vi "main(Test DQMH modules).vi"() -> ()   [LabVIEW 2018, in "Application.lvlib"] (continued)
        n3446 = Not(x=w8018) -> (.not. x?=w8015:bool)
        n3447 = Or(x=w8017, y=w8015) -> (x .or. y?=w8016:bool)
        n3448 = case shown="False" w8016 {
          tunnel: [w8045 _] -> w8027
          tunnel: w8024 -> [w8044 _]
          frame False {
            w8033 = T9 {"command"="", "data"=variant} ("element")
            w8032 = "MEAS.mux6_1"
            n3449 = To Variant(anything=T2."mux6_1_channel3_3" ("mux6_1(3wires)_encode")) -> (Variant=w8042:variant)
            n3450 = To Variant(anything=T2."mux6_1_channel3_2" ("mux6_1(3wires)_encode")) -> (Variant=w8040:variant)
            n3451 = Bundle By Name(cluster=w8033, "command"=w8032, "data"=w8040) -> (w8039:T9)
            n3452 = Bundle By Name(cluster=w8033, "command"=w8032, "data"=w8042) -> (w8038:T9)
            n3453 = Bundle By Name(cluster=w8033, "command"="MEAS.DMM dual read") -> (w8036:T9)
            n3454 = Build Array(w8039, w8038, w8036) -> (w8034:T9[])
            n3455 = Reverse 1D Array(array=w8034) -> (reversed array=w8035:T9[])
            n3456 = for {
              tunnel: [w8051] -> w8045 mode=indexing
              tunnel: w8044 -> [w8050]
              tunnel: w8035 -> [w8049] mode=indexing
              n3457 = Unbundle By Name(w8049) -> ("command"=w8048:string, "data"=w8047:variant)
              n3458 = call "App enquece.vi"("Priority Enquece"=TRUE, "command data"=w8047, "command"=w8048, "queue in"=w8050) -> ("error out"=w8051:errorcluster)  [unwired: 6 in, 1 out]
            }
          }
          frame True {
          }
        }
        n3459 = Merge Errors(w8025, w8027) -> (w8026:errorcluster)
      }
      frame "Test DRV 16" {
        w8061 = 16  # DUT index(1-60)
        n3460 = disable-structure shown="LOGGING==TRUE" {
          disable-tunnel: w8062 -> [w8094 _]
          frame condition #0 (active) {
            n3461 = Empty String/Path?(string/path=w8094) -> (empty?=w8096:bool)
            n3462 = Select(t="Quece timeout", s=w8096, f=w8094) -> (s? t:f=w8093:string)
            n3463 = call "string log (SubVI).vi"("state Name"=w8093) -> ()  [unwired: 9 in, 2 out]
          }
          frame condition #1 {
          }
        }
        n3464 = call "progress string(SubVI).vi"("String 3"=w8062, "String in"=w8063) -> ("String out"=w8064:string)  [unwired: 9 in]
        n3465 = call "FGV DRV stand.vi"() -> ("Sub-Test.DCV"=w8060:bool)  [unwired: 10 in, 1 out]
        n3466 = call "FGV Driver Data.vi"("DUT index(1-60)"=w8061) -> ("DUT SC"=w8059:bool)  [unwired: 7 in, 3 out]
        n3467 = Not(x=w8060) -> (.not. x?=w8056:bool)
        n3468 = Or(x=w8059, y=w8056) -> (x .or. y?=w8058:bool)
        n3469 = case shown="False" w8058 {
          tunnel: [w8086 _] -> w8068
          tunnel: w8066 -> [w8085 _]
          frame False {
            w8074 = T9 {"command"="", "data"=variant} ("element")
            w8073 = "MEAS.mux6_1"
            n3470 = To Variant(anything=T2."mux6_1_channel4_3" ("mux6_1(3wires)_encode")) -> (Variant=w8083:variant)
            n3471 = To Variant(anything=T2."mux6_1_channel4_2" ("mux6_1(3wires)_encode")) -> (Variant=w8081:variant)
            n3472 = Bundle By Name(cluster=w8074, "command"=w8073, "data"=w8081) -> (w8080:T9)
            n3473 = Bundle By Name(cluster=w8074, "command"=w8073, "data"=w8083) -> (w8079:T9)
            n3474 = Bundle By Name(cluster=w8074, "command"="MEAS.DMM dual read") -> (w8077:T9)
            n3475 = Build Array(w8080, w8079, w8077) -> (w8075:T9[])
            n3476 = Reverse 1D Array(array=w8075) -> (reversed array=w8076:T9[])
            n3477 = for {
              tunnel: [w8092] -> w8086 mode=indexing
              tunnel: w8085 -> [w8091]
              tunnel: w8076 -> [w8090] mode=indexing
              n3478 = Unbundle By Name(w8090) -> ("command"=w8089:string, "data"=w8088:variant)
              n3479 = call "App enquece.vi"("Priority Enquece"=TRUE, "command data"=w8088, "command"=w8089, "queue in"=w8091) -> ("error out"=w8092:errorcluster)  [unwired: 6 in, 1 out]
            }
          }
          frame True {
          }
        }
        n3480 = Merge Errors(w8067, w8068) -> (w8057:errorcluster)
      }
      frame "Test DRV 17" {
        w8101 = 17  # DUT index(1-60)
        n3481 = disable-structure shown="LOGGING==TRUE" {
          disable-tunnel: w8102 -> [w8135 _]
          frame condition #0 (active) {
            n3482 = Empty String/Path?(string/path=w8135) -> (empty?=w8137:bool)
            n3483 = Select(t="Quece timeout", s=w8137, f=w8135) -> (s? t:f=w8134:string)
            n3484 = call "string log (SubVI).vi"("state Name"=w8134) -> ()  [unwired: 9 in, 2 out]
          }
          frame condition #1 {
          }
        }
        n3485 = call "progress string(SubVI).vi"("String 3"=w8102, "String in"=w8103) -> ("String out"=w8104:string)  [unwired: 9 in]
        n3486 = call "FGV DRV stand.vi"() -> ("Sub-Test.DCV"=w8100:bool)  [unwired: 10 in, 1 out]
        n3487 = call "FGV Driver Data.vi"("DUT index(1-60)"=w8101) -> ("DUT SC"=w8099:bool)  [unwired: 7 in, 3 out]
        n3488 = Not(x=w8100) -> (.not. x?=w8097:bool)
        n3489 = Or(x=w8099, y=w8097) -> (x .or. y?=w8098:bool)
        n3490 = case shown="False" w8098 {
          tunnel: [w8127 _] -> w8109
          tunnel: w8106 -> [w8126 _]
          frame False {
            w8115 = T9 {"command"="", "data"=variant} ("element")
            w8114 = "MEAS.mux6_1"
            n3491 = To Variant(anything=T2."mux6_1_channel5_3" ("mux6_1(3wires)_encode")) -> (Variant=w8124:variant)
            n3492 = To Variant(anything=T2."mux6_1_channel5_2" ("mux6_1(3wires)_encode")) -> (Variant=w8122:variant)
            n3493 = Bundle By Name(cluster=w8115, "command"=w8114, "data"=w8122) -> (w8121:T9)
            n3494 = Bundle By Name(cluster=w8115, "command"=w8114, "data"=w8124) -> (w8120:T9)
            n3495 = Bundle By Name(cluster=w8115, "command"="MEAS.DMM dual read") -> (w8118:T9)
            n3496 = Build Array(w8121, w8120, w8118) -> (w8116:T9[])
            n3497 = Reverse 1D Array(array=w8116) -> (reversed array=w8117:T9[])
            n3498 = for {
              tunnel: [w8133] -> w8127 mode=indexing
              tunnel: w8126 -> [w8132]
              tunnel: w8117 -> [w8131] mode=indexing
              n3499 = Unbundle By Name(w8131) -> ("command"=w8130:string, "data"=w8129:variant)
              n3500 = call "App enquece.vi"("Priority Enquece"=TRUE, "command data"=w8129, "command"=w8130, "queue in"=w8132) -> ("error out"=w8133:errorcluster)  [unwired: 6 in, 1 out]
            }
          }
          frame True {
          }
        }
        n3501 = Merge Errors(w8107, w8109) -> (w8108:errorcluster)
      }
      frame "Test DRV 18" {
        w8145 = 18  # DUT index(1-60)
        n3502 = disable-structure shown="LOGGING==TRUE" {
          disable-tunnel: w8142 -> [w8176 _]
          frame condition #0 (active) {
            n3503 = Empty String/Path?(string/path=w8176) -> (empty?=w8178:bool)
            n3504 = Select(t="Quece timeout", s=w8178, f=w8176) -> (s? t:f=w8175:string)
            n3505 = call "string log (SubVI).vi"("state Name"=w8175) -> ()  [unwired: 9 in, 2 out]
          }
          frame condition #1 {
          }
        }
        n3506 = call "progress string(SubVI).vi"("String 3"=w8142, "String in"=w8143) -> ("String out"=w8144:string)  [unwired: 9 in]
        n3507 = call "FGV DRV stand.vi"() -> ("Sub-Test.DCV"=w8139:bool)  [unwired: 10 in, 1 out]
        n3508 = call "FGV Driver Data.vi"("DUT index(1-60)"=w8145) -> ("DUT SC"=w8140:bool)  [unwired: 7 in, 3 out]
        n3509 = Not(x=w8139) -> (.not. x?=w8138:bool)
        n3510 = Or(x=w8140, y=w8138) -> (x .or. y?=w8141:bool)
        n3511 = case shown="False" w8141 {
          tunnel: [w8168 _] -> w8150
          tunnel: w8147 -> [w8167 _]
          frame False {
            w8156 = T9 {"command"="", "data"=variant} ("element")
            w8155 = "MEAS.mux6_1"
            n3512 = To Variant(anything=T2."mux6_1_channel6_3" ("mux6_1(3wires)_encode")) -> (Variant=w8165:variant)
            n3513 = To Variant(anything=T2."mux6_1_channel6_2" ("mux6_1(3wires)_encode")) -> (Variant=w8163:variant)
            n3514 = Bundle By Name(cluster=w8156, "command"=w8155, "data"=w8163) -> (w8162:T9)
            n3515 = Bundle By Name(cluster=w8156, "command"=w8155, "data"=w8165) -> (w8161:T9)
            n3516 = Bundle By Name(cluster=w8156, "command"="MEAS.DMM dual read") -> (w8159:T9)
            n3517 = Build Array(w8162, w8161, w8159) -> (w8157:T9[])
            n3518 = Reverse 1D Array(array=w8157) -> (reversed array=w8158:T9[])
            n3519 = for {
              tunnel: [w8174] -> w8168 mode=indexing
              tunnel: w8167 -> [w8173]
              tunnel: w8158 -> [w8172] mode=indexing
              n3520 = Unbundle By Name(w8172) -> ("command"=w8171:string, "data"=w8170:variant)
              n3521 = call "App enquece.vi"("Priority Enquece"=TRUE, "command data"=w8170, "command"=w8171, "queue in"=w8173) -> ("error out"=w8174:errorcluster)  [unwired: 6 in, 1 out]
            }
          }
          frame True {
          }
        }
        n3522 = Merge Errors(w8148, w8150) -> (w8149:errorcluster)
      }
      frame "Test DRV 19" {
        w8183 = 19  # DUT index(1-60)
        n3523 = disable-structure shown="LOGGING==TRUE" {
          disable-tunnel: w8184 -> [w8217 _]
          frame condition #0 (active) {
            n3524 = Empty String/Path?(string/path=w8217) -> (empty?=w8219:bool)
            n3525 = Select(t="Quece timeout", s=w8219, f=w8217) -> (s? t:f=w8216:string)
            n3526 = call "string log (SubVI).vi"("state Name"=w8216) -> ()  [unwired: 9 in, 2 out]
          }
          frame condition #1 {
          }
        }
        n3527 = call "progress string(SubVI).vi"("String 3"=w8184, "String in"=w8185) -> ("String out"=w8186:string)  [unwired: 9 in]
        n3528 = call "FGV Driver Data.vi"("DUT index(1-60)"=w8183) -> ("DUT SC"=w8181:bool)  [unwired: 7 in, 3 out]
        n3529 = call "FGV DRV stand.vi"() -> ("Sub-Test.DCV"=w8180:bool)  [unwired: 10 in, 1 out]
        n3530 = Not(x=w8180) -> (.not. x?=w8179:bool)
        n3531 = Or(x=w8181, y=w8179) -> (x .or. y?=w8182:bool)
        n3532 = case shown="False" w8182 {
          tunnel: [w8209 _] -> w8191
          tunnel: w8188 -> [w8208 _]
          frame False {
            w8197 = T9 {"command"="", "data"=variant} ("element")
            w8196 = "MEAS.mux6_1"
            n3533 = To Variant(anything=T2."mux6_1_channel1_3" ("mux6_1(3wires)_encode")) -> (Variant=w8206:variant)
            n3534 = To Variant(anything=T2."mux6-1_channel1_2" ("mux6_1(3wires)_encode")) -> (Variant=w8204:variant)
            n3535 = Bundle By Name(cluster=w8197, "command"=w8196, "data"=w8204) -> (w8203:T9)
            n3536 = Bundle By Name(cluster=w8197, "command"=w8196, "data"=w8206) -> (w8202:T9)
            n3537 = Bundle By Name(cluster=w8197, "command"="MEAS.DMM dual read") -> (w8200:T9)
            n3538 = Build Array(w8203, w8202, w8200) -> (w8198:T9[])
            n3539 = Reverse 1D Array(array=w8198) -> (reversed array=w8199:T9[])
            n3540 = for {
              tunnel: [w8215] -> w8209 mode=indexing
              tunnel: w8208 -> [w8214]
              tunnel: w8199 -> [w8213] mode=indexing
              n3541 = Unbundle By Name(w8213) -> ("command"=w8212:string, "data"=w8211:variant)
              n3542 = call "App enquece.vi"("Priority Enquece"=TRUE, "command data"=w8211, "command"=w8212, "queue in"=w8214) -> ("error out"=w8215:errorcluster)  [unwired: 6 in, 1 out]
            }
          }
          frame True {
          }
        }
        n3543 = Merge Errors(w8189, w8191) -> (w8190:errorcluster)
      }
      frame "Test DRV 20" {
        w8224 = 20  # DUT index(1-60)
        n3544 = call "progress string(SubVI).vi"("String 3"=w8225, "String in"=w8226) -> ("String out"=w8227:string)  [unwired: 9 in]
        n3545 = disable-structure shown="LOGGING==TRUE" {
          disable-tunnel: w8225 -> [w8258 _]
          frame condition #0 (active) {
            n3546 = Empty String/Path?(string/path=w8258) -> (empty?=w8260:bool)
            n3547 = Select(t="Quece timeout", s=w8260, f=w8258) -> (s? t:f=w8257:string)
            n3548 = call "string log (SubVI).vi"("state Name"=w8257) -> ()  [unwired: 9 in, 2 out]
          }
          frame condition #1 {
          }
        }
        n3549 = call "FGV DRV stand.vi"() -> ("Sub-Test.DCV"=w8223:bool)  [unwired: 10 in, 1 out]
        n3550 = call "FGV Driver Data.vi"("DUT index(1-60)"=w8224) -> ("DUT SC"=w8222:bool)  [unwired: 7 in, 3 out]
        n3551 = Not(x=w8223) -> (.not. x?=w8220:bool)
        n3552 = Or(x=w8222, y=w8220) -> (x .or. y?=w8221:bool)
        n3553 = case shown="False" w8221 {
          tunnel: [w8250 _] -> w8232
          tunnel: w8229 -> [w8249 _]
          frame False {
            w8238 = T9 {"command"="", "data"=variant} ("element")
            w8237 = "MEAS.mux6_1"
            n3554 = To Variant(anything=T2."mux6_1_channel2_3" ("mux6_1(3wires)_encode")) -> (Variant=w8247:variant)
            n3555 = To Variant(anything=T2."mux6_1_channel2_2" ("mux6_1(3wires)_encode")) -> (Variant=w8245:variant)
            n3556 = Bundle By Name(cluster=w8238, "command"=w8237, "data"=w8245) -> (w8244:T9)
            n3557 = Bundle By Name(cluster=w8238, "command"=w8237, "data"=w8247) -> (w8243:T9)
            n3558 = Bundle By Name(cluster=w8238, "command"="MEAS.DMM dual read") -> (w8241:T9)
            n3559 = Build Array(w8244, w8243, w8241) -> (w8239:T9[])
            n3560 = Reverse 1D Array(array=w8239) -> (reversed array=w8240:T9[])
            n3561 = for {
              tunnel: [w8256] -> w8250 mode=indexing
              tunnel: w8249 -> [w8255]
              tunnel: w8240 -> [w8254] mode=indexing
              n3562 = Unbundle By Name(w8254) -> ("command"=w8253:string, "data"=w8252:variant)
              n3563 = call "App enquece.vi"("Priority Enquece"=TRUE, "command data"=w8252, "command"=w8253, "queue in"=w8255) -> ("error out"=w8256:errorcluster)  [unwired: 6 in, 1 out]
            }
          }
          frame True {
          }
        }
        n3564 = Merge Errors(w8230, w8232) -> (w8231:errorcluster)
      }
      frame "Test DRV 21" {
        w8266 = 21  # DUT index(1-60)
        n3565 = call "progress string(SubVI).vi"("String 3"=w8267, "String in"=w8268) -> ("String out"=w8269:string)  [unwired: 9 in]
        n3566 = disable-structure shown="LOGGING==TRUE" {
          disable-tunnel: w8267 -> [w8299 _]
          frame condition #0 (active) {
            n3567 = Empty String/Path?(string/path=w8299) -> (empty?=w8301:bool)
            n3568 = Select(t="Quece timeout", s=w8301, f=w8299) -> (s? t:f=w8298:string)
            n3569 = call "string log (SubVI).vi"("state Name"=w8298) -> ()  [unwired: 9 in, 2 out]
          }
          frame condition #1 {
          }
        }
        n3570 = call "FGV DRV stand.vi"() -> ("Sub-Test.DCV"=w8264:bool)  [unwired: 10 in, 1 out]
        n3571 = call "FGV Driver Data.vi"("DUT index(1-60)"=w8266) -> ("DUT SC"=w8263:bool)  [unwired: 7 in, 3 out]
        n3572 = Not(x=w8264) -> (.not. x?=w8261:bool)
        n3573 = Or(x=w8263, y=w8261) -> (x .or. y?=w8262:bool)
        n3574 = case shown="False" w8262 {
          tunnel: [w8291 _] -> w8273
          tunnel: w8271 -> [w8290 _]
          frame False {
            w8279 = T9 {"command"="", "data"=variant} ("element")
            w8278 = "MEAS.mux6_1"
            n3575 = To Variant(anything=T2."mux6_1_channel3_2" ("mux6_1(3wires)_encode")) -> (Variant=w8286:variant)
            n3576 = To Variant(anything=T2."mux6_1_channel3_3" ("mux6_1(3wires)_encode")) -> (Variant=w8288:variant)
            n3577 = Bundle By Name(cluster=w8279, "command"=w8278, "data"=w8286) -> (w8285:T9)
            n3578 = Bundle By Name(cluster=w8279, "command"=w8278, "data"=w8288) -> (w8284:T9)
            n3579 = Bundle By Name(cluster=w8279, "command"="MEAS.DMM dual read") -> (w8282:T9)
            n3580 = Build Array(w8285, w8284, w8282) -> (w8280:T9[])
            n3581 = Reverse 1D Array(array=w8280) -> (reversed array=w8281:T9[])
            n3582 = for {
              tunnel: [w8297] -> w8291 mode=indexing
              tunnel: w8290 -> [w8296]
              tunnel: w8281 -> [w8295] mode=indexing
              n3583 = Unbundle By Name(w8295) -> ("command"=w8294:string, "data"=w8293:variant)
              n3584 = call "App enquece.vi"("Priority Enquece"=TRUE, "command data"=w8293, "command"=w8294, "queue in"=w8296) -> ("error out"=w8297:errorcluster)  [unwired: 6 in, 1 out]
            }
          }
          frame True {
          }
        }
        n3585 = Merge Errors(w8272, w8273) -> (w8265:errorcluster)
      }
      frame "Test DRV 22" {
        w8306 = 22  # DUT index(1-60)
        n3586 = disable-structure shown="LOGGING==TRUE" {
          disable-tunnel: w8307 -> [w8340 _]
          frame condition #0 (active) {
            n3587 = Empty String/Path?(string/path=w8340) -> (empty?=w8342:bool)
            n3588 = Select(t="Quece timeout", s=w8342, f=w8340) -> (s? t:f=w8339:string)
            n3589 = call "string log (SubVI).vi"("state Name"=w8339) -> ()  [unwired: 9 in, 2 out]
          }
          frame condition #1 {
          }
        }
        n3590 = call "progress string(SubVI).vi"("String 3"=w8307, "String in"=w8308) -> ("String out"=w8309:string)  [unwired: 9 in]
        n3591 = call "FGV DRV stand.vi"() -> ("Sub-Test.DCV"=w8305:bool)  [unwired: 10 in, 1 out]
        n3592 = call "FGV Driver Data.vi"("DUT index(1-60)"=w8306) -> ("DUT SC"=w8304:bool)  [unwired: 7 in, 3 out]
        n3593 = Not(x=w8305) -> (.not. x?=w8302:bool)
        n3594 = Or(x=w8304, y=w8302) -> (x .or. y?=w8303:bool)
        n3595 = case shown="False" w8303 {
          tunnel: [w8332 _] -> w8314
          tunnel: w8311 -> [w8331 _]
          frame False {
            w8320 = T9 {"command"="", "data"=variant} ("element")
            w8319 = "MEAS.mux6_1"
            n3596 = To Variant(anything=T2."mux6_1_channel4_2" ("mux6_1(3wires)_encode")) -> (Variant=w8327:variant)
            n3597 = To Variant(anything=T2."mux6_1_channel4_3" ("mux6_1(3wires)_encode")) -> (Variant=w8329:variant)
            n3598 = Bundle By Name(cluster=w8320, "command"=w8319, "data"=w8327) -> (w8326:T9)
            n3599 = Bundle By Name(cluster=w8320, "command"=w8319, "data"=w8329) -> (w8325:T9)
            n3600 = Bundle By Name(cluster=w8320, "command"="MEAS.DMM dual read") -> (w8323:T9)
            n3601 = Build Array(w8326, w8325, w8323) -> (w8321:T9[])
            n3602 = Reverse 1D Array(array=w8321) -> (reversed array=w8322:T9[])
            n3603 = for {
              tunnel: [w8338] -> w8332 mode=indexing
              tunnel: w8331 -> [w8337]
              tunnel: w8322 -> [w8336] mode=indexing
              n3604 = Unbundle By Name(w8336) -> ("command"=w8335:string, "data"=w8334:variant)
              n3605 = call "App enquece.vi"("Priority Enquece"=TRUE, "command data"=w8334, "command"=w8335, "queue in"=w8337) -> ("error out"=w8338:errorcluster)  [unwired: 6 in, 1 out]
            }
          }
          frame True {
          }
        }
        n3606 = Merge Errors(w8312, w8314) -> (w8313:errorcluster)
      }
      frame "Test DRV 23" {
        w8348 = 23  # DUT index(1-60)
        n3607 = call "progress string(SubVI).vi"("String 3"=w8349, "String in"=w8350) -> ("String out"=w8351:string)  [unwired: 9 in]
        n3608 = disable-structure shown="LOGGING==TRUE" {
          disable-tunnel: w8349 -> [w8381 _]
          frame condition #0 (active) {
            n3609 = Empty String/Path?(string/path=w8381) -> (empty?=w8383:bool)
            n3610 = Select(t="Quece timeout", s=w8383, f=w8381) -> (s? t:f=w8380:string)
            n3611 = call "string log (SubVI).vi"("state Name"=w8380) -> ()  [unwired: 9 in, 2 out]
          }
          frame condition #1 {
          }
        }
        n3612 = call "FGV DRV stand.vi"() -> ("Sub-Test.DCV"=w8346:bool)  [unwired: 10 in, 1 out]
        n3613 = call "FGV Driver Data.vi"("DUT index(1-60)"=w8348) -> ("DUT SC"=w8345:bool)  [unwired: 7 in, 3 out]
        n3614 = Not(x=w8346) -> (.not. x?=w8343:bool)
        n3615 = Or(x=w8345, y=w8343) -> (x .or. y?=w8344:bool)
        n3616 = case shown="False" w8344 {
          tunnel: [w8373 _] -> w8355
          tunnel: w8353 -> [w8372 _]
          frame False {
            w8361 = T9 {"command"="", "data"=variant} ("element")
            w8360 = "MEAS.mux6_1"
            n3617 = To Variant(anything=T2."mux6_1_channel5_3" ("mux6_1(3wires)_encode")) -> (Variant=w8370:variant)
            n3618 = To Variant(anything=T2."mux6_1_channel5_2" ("mux6_1(3wires)_encode")) -> (Variant=w8368:variant)
            n3619 = Bundle By Name(cluster=w8361, "command"=w8360, "data"=w8368) -> (w8367:T9)
            n3620 = Bundle By Name(cluster=w8361, "command"=w8360, "data"=w8370) -> (w8366:T9)
            n3621 = Bundle By Name(cluster=w8361, "command"="MEAS.DMM dual read") -> (w8364:T9)
            n3622 = Build Array(w8367, w8366, w8364) -> (w8362:T9[])
            n3623 = Reverse 1D Array(array=w8362) -> (reversed array=w8363:T9[])
            n3624 = for {
              tunnel: [w8379] -> w8373 mode=indexing
              tunnel: w8372 -> [w8378]
              tunnel: w8363 -> [w8377] mode=indexing
              n3625 = Unbundle By Name(w8377) -> ("command"=w8376:string, "data"=w8375:variant)
              n3626 = call "App enquece.vi"("Priority Enquece"=TRUE, "command data"=w8375, "command"=w8376, "queue in"=w8378) -> ("error out"=w8379:errorcluster)  [unwired: 6 in, 1 out]
            }
          }
          frame True {
          }
        }
        n3627 = Merge Errors(w8354, w8355) -> (w8347:errorcluster)
      }
      frame "Test DRV 24" {
        w8388 = 24  # DUT index(1-60)
        n3628 = call "progress string(SubVI).vi"("String 3"=w8389, "String in"=w8390) -> ("String out"=w8391:string)  [unwired: 9 in]
        n3629 = disable-structure shown="LOGGING==TRUE" {
          disable-tunnel: w8389 -> [w8422 _]
          frame condition #0 (active) {
            n3630 = Empty String/Path?(string/path=w8422) -> (empty?=w8424:bool)
            n3631 = Select(t="Quece timeout", s=w8424, f=w8422) -> (s? t:f=w8421:string)
            n3632 = call "string log (SubVI).vi"("state Name"=w8421) -> ()  [unwired: 9 in, 2 out]
          }
          frame condition #1 {
          }
        }
        n3633 = call "FGV DRV stand.vi"() -> ("Sub-Test.DCV"=w8387:bool)  [unwired: 10 in, 1 out]
        n3634 = Not(x=w8387) -> (.not. x?=w8384:bool)
        n3635 = call "FGV Driver Data.vi"("DUT index(1-60)"=w8388) -> ("DUT SC"=w8386:bool)  [unwired: 7 in, 3 out]
        n3636 = Or(x=w8386, y=w8384) -> (x .or. y?=w8385:bool)
        n3637 = case shown="False" w8385 {
          tunnel: [w8414 _] -> w8396
          tunnel: w8393 -> [w8413 _]
          frame False {
            w8402 = T9 {"command"="", "data"=variant} ("element")
            w8401 = "MEAS.mux6_1"
            n3638 = To Variant(anything=T2."mux6_1_channel6_3" ("mux6_1(3wires)_encode")) -> (Variant=w8411:variant)
            n3639 = To Variant(anything=T2."mux6_1_channel6_2" ("mux6_1(3wires)_encode")) -> (Variant=w8409:variant)
            n3640 = Bundle By Name(cluster=w8402, "command"=w8401, "data"=w8409) -> (w8408:T9)
            n3641 = Bundle By Name(cluster=w8402, "command"=w8401, "data"=w8411) -> (w8407:T9)
            n3642 = Bundle By Name(cluster=w8402, "command"="MEAS.DMM dual read") -> (w8405:T9)
            n3643 = Build Array(w8408, w8407, w8405) -> (w8403:T9[])
            n3644 = Reverse 1D Array(array=w8403) -> (reversed array=w8404:T9[])
            n3645 = for {
              tunnel: [w8420] -> w8414 mode=indexing
              tunnel: w8413 -> [w8419]
              tunnel: w8404 -> [w8418] mode=indexing
              n3646 = Unbundle By Name(w8418) -> ("command"=w8417:string, "data"=w8416:variant)
              n3647 = call "App enquece.vi"("Priority Enquece"=TRUE, "command data"=w8416, "command"=w8417, "queue in"=w8419) -> ("error out"=w8420:errorcluster)  [unwired: 6 in, 1 out]
            }
          }
          frame True {
          }
        }
        n3648 = Merge Errors(w8394, w8396) -> (w8395:errorcluster)
      }
      frame "Test DRV 25" {
        w8429 = 25  # DUT index(1-60)
        n3649 = disable-structure shown="LOGGING==TRUE" {
          disable-tunnel: w8430 -> [w8463 _]
          frame condition #0 (active) {
            n3650 = Empty String/Path?(string/path=w8463) -> (empty?=w8465:bool)
            n3651 = Select(t="Quece timeout", s=w8465, f=w8463) -> (s? t:f=w8462:string)
            n3652 = call "string log (SubVI).vi"("state Name"=w8462) -> ()  [unwired: 9 in, 2 out]
          }
          frame condition #1 {
          }
        }
        n3653 = call "progress string(SubVI).vi"("String 3"=w8430, "String in"=w8431) -> ("String out"=w8432:string)  [unwired: 9 in]
        n3654 = call "FGV DRV stand.vi"() -> ("Sub-Test.DCV"=w8428:bool)  [unwired: 10 in, 1 out]
        n3655 = call "FGV Driver Data.vi"("DUT index(1-60)"=w8429) -> ("DUT SC"=w8427:bool)  [unwired: 7 in, 3 out]
        n3656 = Not(x=w8428) -> (.not. x?=w8425:bool)
        n3657 = Or(x=w8427, y=w8425) -> (x .or. y?=w8426:bool)
        n3658 = case shown="False" w8426 {
          tunnel: [w8455 _] -> w8437
          tunnel: w8434 -> [w8454 _]
          frame False {
            w8443 = T9 {"command"="", "data"=variant} ("element")
            w8442 = "MEAS.mux6_1"
            n3659 = To Variant(anything=T2."mux6_1_channel1_3" ("mux6_1(3wires)_encode")) -> (Variant=w8452:variant)
            n3660 = To Variant(anything=T2."mux6-1_channel1_2" ("mux6_1(3wires)_encode")) -> (Variant=w8450:variant)
            n3661 = Bundle By Name(cluster=w8443, "command"=w8442, "data"=w8450) -> (w8449:T9)
            n3662 = Bundle By Name(cluster=w8443, "command"=w8442, "data"=w8452) -> (w8448:T9)
            n3663 = Bundle By Name(cluster=w8443, "command"="MEAS.DMM dual read") -> (w8446:T9)
            n3664 = Build Array(w8449, w8448, w8446) -> (w8444:T9[])
            n3665 = Reverse 1D Array(array=w8444) -> (reversed array=w8445:T9[])
            n3666 = for {
              tunnel: [w8461] -> w8455 mode=indexing
              tunnel: w8454 -> [w8460]
              tunnel: w8445 -> [w8456] mode=indexing
              n3667 = Unbundle By Name(w8456) -> ("command"=w8459:string, "data"=w8458:variant)
              n3668 = call "App enquece.vi"("Priority Enquece"=TRUE, "command data"=w8458, "command"=w8459, "queue in"=w8460) -> ("error out"=w8461:errorcluster)  [unwired: 6 in, 1 out]
            }
          }
          frame True {
          }
        }
        n3669 = Merge Errors(w8435, w8437) -> (w8436:errorcluster)
      }
      frame "Test DRV 26" {
        w8471 = 26  # DUT index(1-60)
        n3670 = disable-structure shown="LOGGING==TRUE" {
          disable-tunnel: w8472 -> [w8504 _]
          frame condition #0 (active) {
            n3671 = Empty String/Path?(string/path=w8504) -> (empty?=w8506:bool)
            n3672 = Select(t="Quece timeout", s=w8506, f=w8504) -> (s? t:f=w8503:string)
            n3673 = call "string log (SubVI).vi"("state Name"=w8503) -> ()  [unwired: 9 in, 2 out]
          }
          frame condition #1 {
          }
        }
        n3674 = call "progress string(SubVI).vi"("String 3"=w8472, "String in"=w8473) -> ("String out"=w8474:string)  [unwired: 9 in]
        n3675 = call "FGV DRV stand.vi"() -> ("Sub-Test.DCV"=w8469:bool)  [unwired: 10 in, 1 out]
        n3676 = call "FGV Driver Data.vi"("DUT index(1-60)"=w8471) -> ("DUT SC"=w8468:bool)  [unwired: 7 in, 3 out]
        n3677 = Not(x=w8469) -> (.not. x?=w8466:bool)
        n3678 = Or(x=w8468, y=w8466) -> (x .or. y?=w8467:bool)
        n3679 = case shown="False" w8467 {
          tunnel: [w8496 _] -> w8478
          tunnel: w8476 -> [w8495 _]
          frame False {
            w8484 = T9 {"command"="", "data"=variant} ("element")
            w8483 = "MEAS.mux6_1"
            n3680 = To Variant(anything=T2."mux6_1_channel2_3" ("mux6_1(3wires)_encode")) -> (Variant=w8493:variant)
            n3681 = To Variant(anything=T2."mux6_1_channel2_2" ("mux6_1(3wires)_encode")) -> (Variant=w8491:variant)
            n3682 = Bundle By Name(cluster=w8484, "command"=w8483, "data"=w8491) -> (w8490:T9)
            n3683 = Bundle By Name(cluster=w8484, "command"=w8483, "data"=w8493) -> (w8489:T9)
            n3684 = Bundle By Name(cluster=w8484, "command"="MEAS.DMM dual read") -> (w8487:T9)
            n3685 = Build Array(w8490, w8489, w8487) -> (w8485:T9[])
            n3686 = Reverse 1D Array(array=w8485) -> (reversed array=w8486:T9[])
            n3687 = for {
              tunnel: [w8502] -> w8496 mode=indexing
              tunnel: w8495 -> [w8501]
              tunnel: w8486 -> [w8500] mode=indexing
              n3688 = Unbundle By Name(w8500) -> ("command"=w8499:string, "data"=w8498:variant)
              n3689 = call "App enquece.vi"("Priority Enquece"=TRUE, "command data"=w8498, "command"=w8499, "queue in"=w8501) -> ("error out"=w8502:errorcluster)  [unwired: 6 in, 1 out]
            }
          }
          frame True {
          }
        }
        n3690 = Merge Errors(w8477, w8478) -> (w8470:errorcluster)
      }
      frame "Test DRV 27" {
        w8511 = 27  # DUT index(1-60)
        n3691 = disable-structure shown="LOGGING==TRUE" {
          disable-tunnel: w8512 -> [w8545 _]
          frame condition #0 (active) {
            n3692 = Empty String/Path?(string/path=w8545) -> (empty?=w8547:bool)
            n3693 = Select(t="Quece timeout", s=w8547, f=w8545) -> (s? t:f=w8544:string)
            n3694 = call "string log (SubVI).vi"("state Name"=w8544) -> ()  [unwired: 9 in, 2 out]
          }
          frame condition #1 {
          }
        }
        n3695 = call "progress string(SubVI).vi"("String 3"=w8512, "String in"=w8513) -> ("String out"=w8514:string)  [unwired: 9 in]
        n3696 = call "FGV DRV stand.vi"() -> ("Sub-Test.DCV"=w8510:bool)  [unwired: 10 in, 1 out]
        n3697 = call "FGV Driver Data.vi"("DUT index(1-60)"=w8511) -> ("DUT SC"=w8509:bool)  [unwired: 7 in, 3 out]
        n3698 = Not(x=w8510) -> (.not. x?=w8507:bool)
        n3699 = Or(x=w8509, y=w8507) -> (x .or. y?=w8508:bool)
        n3700 = case shown="False" w8508 {
          tunnel: [w8537 _] -> w8519
          tunnel: w8516 -> [w8536 _]
          frame False {
            w8525 = T9 {"command"="", "data"=variant} ("element")
            w8524 = "MEAS.mux6_1"
            n3701 = To Variant(anything=T2."mux6_1_channel3_3" ("mux6_1(3wires)_encode")) -> (Variant=w8534:variant)
            n3702 = To Variant(anything=T2."mux6_1_channel3_2" ("mux6_1(3wires)_encode")) -> (Variant=w8532:variant)
            n3703 = Bundle By Name(cluster=w8525, "command"=w8524, "data"=w8532) -> (w8531:T9)
            n3704 = Bundle By Name(cluster=w8525, "command"=w8524, "data"=w8534) -> (w8530:T9)
            n3705 = Bundle By Name(cluster=w8525, "command"="MEAS.DMM dual read") -> (w8528:T9)
            n3706 = Build Array(w8531, w8530, w8528) -> (w8526:T9[])
            n3707 = Reverse 1D Array(array=w8526) -> (reversed array=w8527:T9[])
            n3708 = for {
              tunnel: [w8543] -> w8537 mode=indexing
              tunnel: w8536 -> [w8542]
              tunnel: w8527 -> [w8541] mode=indexing
              n3709 = Unbundle By Name(w8541) -> ("command"=w8540:string, "data"=w8539:variant)
              n3710 = call "App enquece.vi"("Priority Enquece"=TRUE, "command data"=w8539, "command"=w8540, "queue in"=w8542) -> ("error out"=w8543:errorcluster)  [unwired: 6 in, 1 out]
            }
          }
          frame True {
          }
        }
        n3711 = Merge Errors(w8517, w8519) -> (w8518:errorcluster)
      }
      frame "Test DRV 28" {
        w8552 = 28  # DUT index(1-60)
        n3712 = disable-structure shown="LOGGING==TRUE" {
          disable-tunnel: w8553 -> [w8586 _]
          frame condition #0 (active) {
            n3713 = Empty String/Path?(string/path=w8586) -> (empty?=w8588:bool)
            n3714 = Select(t="Quece timeout", s=w8588, f=w8586) -> (s? t:f=w8585:string)
            n3715 = call "string log (SubVI).vi"("state Name"=w8585) -> ()  [unwired: 9 in, 2 out]
          }
          frame condition #1 {
          }
        }
        n3716 = call "progress string(SubVI).vi"("String 3"=w8553, "String in"=w8554) -> ("String out"=w8555:string)  [unwired: 9 in]
        n3717 = call "FGV DRV stand.vi"() -> ("Sub-Test.DCV"=w8551:bool)  [unwired: 10 in, 1 out]
        n3718 = call "FGV Driver Data.vi"("DUT index(1-60)"=w8552) -> ("DUT SC"=w8550:bool)  [unwired: 7 in, 3 out]
        n3719 = Not(x=w8551) -> (.not. x?=w8548:bool)
        n3720 = Or(x=w8550, y=w8548) -> (x .or. y?=w8549:bool)
        n3721 = case shown="False" w8549 {
          tunnel: [w8578 _] -> w8560
          tunnel: w8557 -> [w8577 _]
          frame False {
            w8565 = T9 {"command"="", "data"=variant} ("element")
            w8566 = "MEAS.mux6_1"
            n3722 = To Variant(anything=T2."mux6_1_channel4_3" ("mux6_1(3wires)_encode")) -> (Variant=w8575:variant)
            n3723 = To Variant(anything=T2."mux6_1_channel4_2" ("mux6_1(3wires)_encode")) -> (Variant=w8573:variant)
            n3724 = Bundle By Name(cluster=w8565, "command"=w8566, "data"=w8573) -> (w8572:T9)
            n3725 = Bundle By Name(cluster=w8565, "command"=w8566, "data"=w8575) -> (w8571:T9)
            n3726 = Bundle By Name(cluster=w8565, "command"="MEAS.DMM dual read") -> (w8569:T9)
            n3727 = Build Array(w8572, w8571, w8569) -> (w8567:T9[])
            n3728 = Reverse 1D Array(array=w8567) -> (reversed array=w8568:T9[])
            n3729 = for {
              tunnel: [w8584] -> w8578 mode=indexing
              tunnel: w8577 -> [w8583]
              tunnel: w8568 -> [w8582] mode=indexing
              n3730 = Unbundle By Name(w8582) -> ("command"=w8581:string, "data"=w8580:variant)
              n3731 = call "App enquece.vi"("Priority Enquece"=TRUE, "command data"=w8580, "command"=w8581, "queue in"=w8583) -> ("error out"=w8584:errorcluster)  [unwired: 6 in, 1 out]
            }
          }
          frame True {
          }
        }
        n3732 = Merge Errors(w8558, w8560) -> (w8559:errorcluster)
      }
      frame "Test DRV 29" {
        w8593 = 29  # DUT index(1-60)
        n3733 = disable-structure shown="LOGGING==TRUE" {
          disable-tunnel: w8594 -> [w8627 _]
          frame condition #0 (active) {
            n3734 = Empty String/Path?(string/path=w8627) -> (empty?=w8629:bool)
            n3735 = Select(t="Quece timeout", s=w8629, f=w8627) -> (s? t:f=w8626:string)
            n3736 = call "string log (SubVI).vi"("state Name"=w8626) -> ()  [unwired: 9 in, 2 out]
          }
          frame condition #1 {
          }
        }
        n3737 = call "progress string(SubVI).vi"("String 3"=w8594, "String in"=w8595) -> ("String out"=w8596:string)  [unwired: 9 in]
        n3738 = call "FGV DRV stand.vi"() -> ("Sub-Test.DCV"=w8592:bool)  [unwired: 10 in, 1 out]
        n3739 = call "FGV Driver Data.vi"("DUT index(1-60)"=w8593) -> ("DUT SC"=w8591:bool)  [unwired: 7 in, 3 out]
        n3740 = Not(x=w8592) -> (.not. x?=w8589:bool)
        n3741 = Or(x=w8591, y=w8589) -> (x .or. y?=w8590:bool)
        n3742 = case shown="False" w8590 {
          tunnel: [w8619 _] -> w8601
          tunnel: w8598 -> [w8618 _]
          frame False {
            w8607 = T9 {"command"="", "data"=variant} ("element")
            w8606 = "MEAS.mux6_1"
            n3743 = To Variant(anything=T2."mux6_1_channel5_3" ("mux6_1(3wires)_encode")) -> (Variant=w8616:variant)
            n3744 = To Variant(anything=T2."mux6_1_channel5_2" ("mux6_1(3wires)_encode")) -> (Variant=w8614:variant)
            n3745 = Bundle By Name(cluster=w8607, "command"=w8606, "data"=w8614) -> (w8613:T9)
            n3746 = Bundle By Name(cluster=w8607, "command"=w8606, "data"=w8616) -> (w8612:T9)
            n3747 = Bundle By Name(cluster=w8607, "command"="MEAS.DMM dual read") -> (w8610:T9)
            n3748 = Build Array(w8613, w8612, w8610) -> (w8608:T9[])
            n3749 = Reverse 1D Array(array=w8608) -> (reversed array=w8609:T9[])
            n3750 = for {
              tunnel: [w8625] -> w8619 mode=indexing
              tunnel: w8618 -> [w8624]
              tunnel: w8609 -> [w8623] mode=indexing
              n3751 = Unbundle By Name(w8623) -> ("command"=w8622:string, "data"=w8621:variant)
              n3752 = call "App enquece.vi"("Priority Enquece"=TRUE, "command data"=w8621, "command"=w8622, "queue in"=w8624) -> ("error out"=w8625:errorcluster)  [unwired: 6 in, 1 out]
            }
          }
          frame True {
          }
        }
        n3753 = Merge Errors(w8599, w8601) -> (w8600:errorcluster)
      }
      frame "Test DRV 30" {
        w8634 = 30  # DUT index(1-60)
        n3754 = disable-structure shown="LOGGING==TRUE" {
          disable-tunnel: w8635 -> [w8668 _]
          frame condition #0 (active) {
            n3755 = Empty String/Path?(string/path=w8668) -> (empty?=w8670:bool)
            n3756 = Select(t="Quece timeout", s=w8670, f=w8668) -> (s? t:f=w8667:string)
            n3757 = call "string log (SubVI).vi"("state Name"=w8667) -> ()  [unwired: 9 in, 2 out]
          }
          frame condition #1 {
          }
        }
        n3758 = call "progress string(SubVI).vi"("String 3"=w8635, "String in"=w8636) -> ("String out"=w8637:string)  [unwired: 9 in]
        n3759 = call "FGV DRV stand.vi"() -> ("Sub-Test.DCV"=w8631:bool)  [unwired: 10 in, 1 out]
        n3760 = call "FGV Driver Data.vi"("DUT index(1-60)"=w8634) -> ("DUT SC"=w8632:bool)  [unwired: 7 in, 3 out]
        n3761 = Not(x=w8631) -> (.not. x?=w8630:bool)
        n3762 = Or(x=w8632, y=w8630) -> (x .or. y?=w8633:bool)
        n3763 = case shown="False" w8633 {
          tunnel: [w8660 _] -> w8642
          tunnel: w8639 -> [w8659 _]
          frame False {
            w8648 = T9 {"command"="", "data"=variant} ("element")
            w8647 = "MEAS.mux6_1"
            n3764 = To Variant(anything=T2."mux6_1_channel6_3" ("mux6_1(3wires)_encode")) -> (Variant=w8657:variant)
            n3765 = To Variant(anything=T2."mux6_1_channel6_2" ("mux6_1(3wires)_encode")) -> (Variant=w8655:variant)
            n3766 = Bundle By Name(cluster=w8648, "command"=w8647, "data"=w8655) -> (w8654:T9)
            n3767 = Bundle By Name(cluster=w8648, "command"=w8647, "data"=w8657) -> (w8653:T9)
            n3768 = Bundle By Name(cluster=w8648, "command"="MEAS.DMM dual read") -> (w8651:T9)
            n3769 = Build Array(w8654, w8653, w8651) -> (w8649:T9[])
            n3770 = Reverse 1D Array(array=w8649) -> (reversed array=w8650:T9[])
            n3771 = for {
              tunnel: [w8666] -> w8660 mode=indexing
              tunnel: w8659 -> [w8665]
              tunnel: w8650 -> [w8664] mode=indexing
              n3772 = Unbundle By Name(w8664) -> ("command"=w8663:string, "data"=w8662:variant)
              n3773 = call "App enquece.vi"("Priority Enquece"=TRUE, "command data"=w8662, "command"=w8663, "queue in"=w8665) -> ("error out"=w8666:errorcluster)  [unwired: 6 in, 1 out]
            }
          }
          frame True {
          }
        }
        n3774 = Merge Errors(w8640, w8642) -> (w8641:errorcluster)
      }
      frame "Test DRV 31" {
        w8675 = 31  # DUT index(1-60)
        n3775 = disable-structure shown="LOGGING==TRUE" {
          disable-tunnel: w8676 -> [w8709 _]
          frame condition #0 (active) {
            n3776 = Empty String/Path?(string/path=w8709) -> (empty?=w8711:bool)
            n3777 = Select(t="Quece timeout", s=w8711, f=w8709) -> (s? t:f=w8708:string)
            n3778 = call "string log (SubVI).vi"("state Name"=w8708) -> ()  [unwired: 9 in, 2 out]
          }
          frame condition #1 {
          }
        }
        n3779 = call "progress string(SubVI).vi"("String 3"=w8676, "String in"=w8677) -> ("String out"=w8678:string)  [unwired: 9 in]
        n3780 = call "FGV DRV stand.vi"() -> ("Sub-Test.DCV"=w8674:bool)  [unwired: 10 in, 1 out]
        n3781 = call "FGV Driver Data.vi"("DUT index(1-60)"=w8675) -> ("DUT SC"=w8673:bool)  [unwired: 7 in, 3 out]
        n3782 = Not(x=w8674) -> (.not. x?=w8671:bool)
        n3783 = Or(x=w8673, y=w8671) -> (x .or. y?=w8672:bool)
        n3784 = case shown="False" w8672 {
          tunnel: [w8701 _] -> w8683
          tunnel: w8680 -> [w8700 _]
          frame False {
            w8689 = T9 {"command"="", "data"=variant} ("element")
            w8688 = "MEAS.mux6_1"
            n3785 = To Variant(anything=T2."mux6_1_channel1_3" ("mux6_1(3wires)_encode")) -> (Variant=w8698:variant)
            n3786 = To Variant(anything=T2."mux6-1_channel1_2" ("mux6_1(3wires)_encode")) -> (Variant=w8696:variant)
            n3787 = Bundle By Name(cluster=w8689, "command"=w8688, "data"=w8696) -> (w8695:T9)
            n3788 = Bundle By Name(cluster=w8689, "command"=w8688, "data"=w8698) -> (w8694:T9)
            n3789 = Bundle By Name(cluster=w8689, "command"="MEAS.DMM dual read") -> (w8692:T9)
            n3790 = Build Array(w8695, w8694, w8692) -> (w8690:T9[])
            n3791 = Reverse 1D Array(array=w8690) -> (reversed array=w8691:T9[])
            n3792 = for {
              tunnel: [w8707] -> w8701 mode=indexing
              tunnel: w8700 -> [w8706]
              tunnel: w8691 -> [w8705] mode=indexing
              n3793 = Unbundle By Name(w8705) -> ("command"=w8704:string, "data"=w8703:variant)
              n3794 = call "App enquece.vi"("Priority Enquece"=TRUE, "command data"=w8703, "command"=w8704, "queue in"=w8706) -> ("error out"=w8707:errorcluster)  [unwired: 6 in, 1 out]
            }
          }
          frame True {
          }
        }
        n3795 = Merge Errors(w8681, w8683) -> (w8682:errorcluster)
      }
      frame "Test DRV 32" {
        w8716 = 32  # DUT index(1-60)
        n3796 = disable-structure shown="LOGGING==TRUE" {
          disable-tunnel: w8717 -> [w8750 _]
          frame condition #0 (active) {
            n3797 = Empty String/Path?(string/path=w8750) -> (empty?=w8752:bool)
            n3798 = Select(t="Quece timeout", s=w8752, f=w8750) -> (s? t:f=w8749:string)
            n3799 = call "string log (SubVI).vi"("state Name"=w8749) -> ()  [unwired: 9 in, 2 out]
          }
          frame condition #1 {
          }
        }
        n3800 = call "progress string(SubVI).vi"("String 3"=w8717, "String in"=w8718) -> ("String out"=w8719:string)  [unwired: 9 in]
        n3801 = call "FGV DRV stand.vi"() -> ("Sub-Test.DCV"=w8715:bool)  [unwired: 10 in, 1 out]
        n3802 = call "FGV Driver Data.vi"("DUT index(1-60)"=w8716) -> ("DUT SC"=w8714:bool)  [unwired: 7 in, 3 out]
        n3803 = Not(x=w8715) -> (.not. x?=w8712:bool)
        n3804 = Or(x=w8714, y=w8712) -> (x .or. y?=w8713:bool)
        n3805 = case shown="False" w8713 {
          tunnel: [w8742 _] -> w8724
          tunnel: w8721 -> [w8741 _]
          frame False {
            w8730 = T9 {"command"="", "data"=variant} ("element")
            w8729 = "MEAS.mux6_1"
            n3806 = To Variant(anything=T2."mux6_1_channel2_3" ("mux6_1(3wires)_encode")) -> (Variant=w8739:variant)
            n3807 = To Variant(anything=T2."mux6_1_channel2_2" ("mux6_1(3wires)_encode")) -> (Variant=w8737:variant)
            n3808 = Bundle By Name(cluster=w8730, "command"=w8729, "data"=w8737) -> (w8736:T9)
            n3809 = Bundle By Name(cluster=w8730, "command"=w8729, "data"=w8739) -> (w8735:T9)
            n3810 = Bundle By Name(cluster=w8730, "command"="MEAS.DMM dual read") -> (w8733:T9)
            n3811 = Build Array(w8736, w8735, w8733) -> (w8731:T9[])
            n3812 = Reverse 1D Array(array=w8731) -> (reversed array=w8732:T9[])
            n3813 = for {
              tunnel: [w8748] -> w8742 mode=indexing
              tunnel: w8741 -> [w8747]
              tunnel: w8732 -> [w8746] mode=indexing
              n3814 = Unbundle By Name(w8746) -> ("command"=w8745:string, "data"=w8744:variant)
              n3815 = call "App enquece.vi"("Priority Enquece"=TRUE, "command data"=w8744, "command"=w8745, "queue in"=w8747) -> ("error out"=w8748:errorcluster)  [unwired: 6 in, 1 out]
            }
          }
          frame True {
          }
        }
        n3816 = Merge Errors(w8722, w8724) -> (w8723:errorcluster)
      }
      frame "Test DRV 33" {
        w8757 = 33  # DUT index(1-60)
        n3817 = call "progress string(SubVI).vi"("String 3"=w8758, "String in"=w8759) -> ("String out"=w8760:string)  [unwired: 9 in]
        n3818 = disable-structure shown="LOGGING==TRUE" {
          disable-tunnel: w8758 -> [w8791 _]
          frame condition #0 (active) {
            n3819 = Empty String/Path?(string/path=w8791) -> (empty?=w8793:bool)
            n3820 = Select(t="Quece timeout", s=w8793, f=w8791) -> (s? t:f=w8790:string)
            n3821 = call "string log (SubVI).vi"("state Name"=w8790) -> ()  [unwired: 9 in, 2 out]
          }
          frame condition #1 {
          }
        }
        n3822 = call "FGV Driver Data.vi"("DUT index(1-60)"=w8757) -> ("DUT SC"=w8755:bool)  [unwired: 7 in, 3 out]
        n3823 = call "FGV DRV stand.vi"() -> ("Sub-Test.DCV"=w8756:bool)  [unwired: 10 in, 1 out]
        n3824 = Not(x=w8756) -> (.not. x?=w8753:bool)
        n3825 = Or(x=w8755, y=w8753) -> (x .or. y?=w8754:bool)
        n3826 = case shown="False" w8754 {
          tunnel: [w8783 _] -> w8765
          tunnel: w8762 -> [w8782 _]
          frame False {
            w8771 = T9 {"command"="", "data"=variant} ("element")
            w8770 = "MEAS.mux6_1"
            n3827 = To Variant(anything=T2."mux6_1_channel3_3" ("mux6_1(3wires)_encode")) -> (Variant=w8780:variant)
            n3828 = To Variant(anything=T2."mux6_1_channel3_2" ("mux6_1(3wires)_encode")) -> (Variant=w8778:variant)
            n3829 = Bundle By Name(cluster=w8771, "command"=w8770, "data"=w8778) -> (w8777:T9)
            n3830 = Bundle By Name(cluster=w8771, "command"=w8770, "data"=w8780) -> (w8776:T9)
            n3831 = Bundle By Name(cluster=w8771, "command"="MEAS.DMM dual read") -> (w8774:T9)
            n3832 = Build Array(w8777, w8776, w8774) -> (w8772:T9[])
            n3833 = Reverse 1D Array(array=w8772) -> (reversed array=w8773:T9[])
            n3834 = for {
              tunnel: [w8789] -> w8783 mode=indexing
              tunnel: w8782 -> [w8788]
              tunnel: w8773 -> [w8787] mode=indexing
              n3835 = Unbundle By Name(w8787) -> ("command"=w8786:string, "data"=w8785:variant)
              n3836 = call "App enquece.vi"("Priority Enquece"=TRUE, "command data"=w8785, "command"=w8786, "queue in"=w8788) -> ("error out"=w8789:errorcluster)  [unwired: 6 in, 1 out]
            }
          }
          frame True {
          }
        }
        n3837 = Merge Errors(w8763, w8765) -> (w8764:errorcluster)
      }
      frame "Test DRV 34" {
        w8799 = 34  # DUT index(1-60)
        n3838 = disable-structure shown="LOGGING==TRUE" {
          disable-tunnel: w8800 -> [w8832 _]
          frame condition #0 (active) {
            n3839 = Empty String/Path?(string/path=w8832) -> (empty?=w8834:bool)
            n3840 = Select(t="Quece timeout", s=w8834, f=w8832) -> (s? t:f=w8831:string)
            n3841 = call "string log (SubVI).vi"("state Name"=w8831) -> ()  [unwired: 9 in, 2 out]
          }
          frame condition #1 {
          }
        }
        n3842 = call "progress string(SubVI).vi"("String 3"=w8800, "String in"=w8801) -> ("String out"=w8802:string)  [unwired: 9 in]
        n3843 = call "FGV DRV stand.vi"() -> ("Sub-Test.DCV"=w8797:bool)  [unwired: 10 in, 1 out]
        n3844 = call "FGV Driver Data.vi"("DUT index(1-60)"=w8799) -> ("DUT SC"=w8796:bool)  [unwired: 7 in, 3 out]
        n3845 = Not(x=w8797) -> (.not. x?=w8794:bool)
        n3846 = Or(x=w8796, y=w8794) -> (x .or. y?=w8795:bool)
        n3847 = case shown="False" w8795 {
          tunnel: [w8824 _] -> w8806
          tunnel: w8804 -> [w8823 _]
          frame False {
            w8812 = T9 {"command"="", "data"=variant} ("element")
            w8811 = "MEAS.mux6_1"
            n3848 = To Variant(anything=T2."mux6_1_channel4_3" ("mux6_1(3wires)_encode")) -> (Variant=w8821:variant)
            n3849 = To Variant(anything=T2."mux6_1_channel4_2" ("mux6_1(3wires)_encode")) -> (Variant=w8819:variant)
            n3850 = Bundle By Name(cluster=w8812, "command"=w8811, "data"=w8819) -> (w8818:T9)
            n3851 = Bundle By Name(cluster=w8812, "command"=w8811, "data"=w8821) -> (w8817:T9)
            n3852 = Bundle By Name(cluster=w8812, "command"="MEAS.DMM dual read") -> (w8815:T9)
            n3853 = Build Array(w8818, w8817, w8815) -> (w8813:T9[])
            n3854 = Reverse 1D Array(array=w8813) -> (reversed array=w8814:T9[])
            n3855 = for {
              tunnel: [w8830] -> w8824 mode=indexing
              tunnel: w8823 -> [w8829]
              tunnel: w8814 -> [w8828] mode=indexing
              n3856 = Unbundle By Name(w8828) -> ("command"=w8827:string, "data"=w8826:variant)
              n3857 = call "App enquece.vi"("Priority Enquece"=TRUE, "command data"=w8826, "command"=w8827, "queue in"=w8829) -> ("error out"=w8830:errorcluster)  [unwired: 6 in, 1 out]
            }
          }
          frame True {
          }
        }
        n3858 = Merge Errors(w8805, w8806) -> (w8798:errorcluster)
      }
      frame "Test DRV 35" {
        w8839 = 35  # DUT index(1-60
        n3859 = disable-structure shown="LOGGING==TRUE" {
          disable-tunnel: w8840 -> [w8873 _]
          frame condition #0 (active) {
            n3860 = Empty String/Path?(string/path=w8873) -> (empty?=w8875:bool)
            n3861 = Select(t="Quece timeout", s=w8875, f=w8873) -> (s? t:f=w8872:string)
            n3862 = call "string log (SubVI).vi"("state Name"=w8872) -> ()  [unwired: 9 in, 2 out]
          }
          frame condition #1 {
          }
        }
        n3863 = call "progress string(SubVI).vi"("String 3"=w8840, "String in"=w8841) -> ("String out"=w8842:string)  [unwired: 9 in]
        n3864 = call "FGV Driver Data.vi"("DUT index(1-60)"=w8839) -> ("DUT SC"=w8837:bool)  [unwired: 7 in, 3 out]
        n3865 = call "FGV DRV stand.vi"() -> ("Sub-Test.DCV"=w8838:bool)  [unwired: 10 in, 1 out]
        n3866 = Not(x=w8838) -> (.not. x?=w8835:bool)
        n3867 = Or(x=w8837, y=w8835) -> (x .or. y?=w8836:bool)
        n3868 = case shown="False" w8836 {
          tunnel: [w8865 _] -> w8847
          tunnel: w8844 -> [w8864 _]
          frame False {
            w8853 = T9 {"command"="", "data"=variant} ("element")
            w8852 = "MEAS.mux6_1"
            n3869 = To Variant(anything=T2."mux6_1_channel5_3" ("mux6_1(3wires)_encode")) -> (Variant=w8862:variant)
            n3870 = To Variant(anything=T2."mux6_1_channel5_2" ("mux6_1(3wires)_encode")) -> (Variant=w8860:variant)
            n3871 = Bundle By Name(cluster=w8853, "command"=w8852, "data"=w8860) -> (w8859:T9)
            n3872 = Bundle By Name(cluster=w8853, "command"=w8852, "data"=w8862) -> (w8858:T9)
            n3873 = Bundle By Name(cluster=w8853, "command"="MEAS.DMM dual read") -> (w8856:T9)
            n3874 = Build Array(w8859, w8858, w8856) -> (w8854:T9[])
            n3875 = Reverse 1D Array(array=w8854) -> (reversed array=w8855:T9[])
            n3876 = for {
              tunnel: [w8871] -> w8865 mode=indexing
              tunnel: w8864 -> [w8870]
              tunnel: w8855 -> [w8869] mode=indexing
              n3877 = Unbundle By Name(w8869) -> ("command"=w8868:string, "data"=w8867:variant)
              n3878 = call "App enquece.vi"("Priority Enquece"=TRUE, "command data"=w8867, "command"=w8868, "queue in"=w8870) -> ("error out"=w8871:errorcluster)  [unwired: 6 in, 1 out]
            }
          }
          frame True {
          }
        }
        n3879 = Merge Errors(w8845, w8847) -> (w8846:errorcluster)
      }
      frame "Test DRV 36" {
        w8880 = 36  # DUT index(1-60)
        n3880 = disable-structure shown="LOGGING==TRUE" {
          disable-tunnel: w8881 -> [w8914 _]
          frame condition #0 (active) {
            n3881 = Empty String/Path?(string/path=w8914) -> (empty?=w8916:bool)
            n3882 = Select(t="Quece timeout", s=w8916, f=w8914) -> (s? t:f=w8913:string)
            n3883 = call "string log (SubVI).vi"("state Name"=w8913) -> ()  [unwired: 9 in, 2 out]
          }
          frame condition #1 {
          }
        }
        n3884 = call "progress string(SubVI).vi"("String 3"=w8881, "String in"=w8882) -> ("String out"=w8883:string)  [unwired: 9 in]
        n3885 = call "FGV DRV stand.vi"() -> ("Sub-Test.DCV"=w8879:bool)  [unwired: 10 in, 1 out]
        n3886 = call "FGV Driver Data.vi"("DUT index(1-60)"=w8880) -> ("DUT SC"=w8878:bool)  [unwired: 7 in, 3 out]
        n3887 = Not(x=w8879) -> (.not. x?=w8876:bool)
